vi "FlatToRichcif_pluginloader_DiscoveredPlugin.vi"(5 "OutputClusterType":T1, 11 "InputCluster":T4) -> (3 "OutputCluster":T1)   [LabVIEW 2021, in "CIF_PluginLoader_server.lvlib"]
uses:
  CIF_PluginLoader_server.lvlib
  cif_pluginloader_DiscoveredPlugin_Flat.ctl
  cif_common_Version_Flat.ctl
  cif_management_common_PluginMetadata_Flat.ctl
  cif_pluginloader_DiscoveredPlugin.ctl
  cif_common_Version.ctl
  cif_management_common_PluginMetadata.ctl
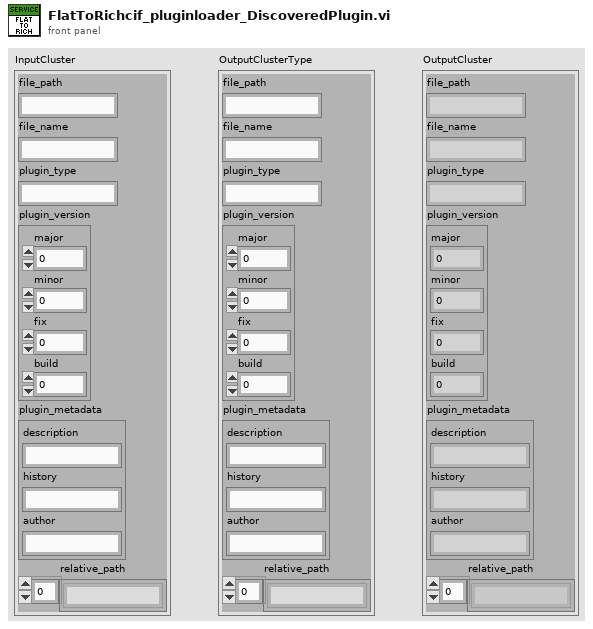
[diagram p1: front panel]
types:
  T1 = typedef "CIF_PluginLoader_server.lvlib/cif_pluginloader_DiscoveredPlugin.ctl" = cluster{"file_path":string, "file_name":string, "plugin_type":string, "plugin_version":T2, "plugin_metadata":T3, "relative_path":string[]}
  T2 = typedef "CIF_PluginLoader_server.lvlib/cif_common_Version.ctl" = cluster{"major":u32, "minor":u32, "fix":u32, "build":u32}
  T3 = typedef "CIF_PluginLoader_server.lvlib/cif_management_common_PluginMetadata.ctl" = cluster{"description":string, "history":string, "author":string}
  T4 = typedef "CIF_PluginLoader_server.lvlib/cif_pluginloader_DiscoveredPlugin_Flat.ctl" = cluster{"file_path":string, "file_name":string, "plugin_type":string, "plugin_version":T5, "plugin_metadata":T6, "relative_path":string[]}
  T5 = typedef "CIF_PluginLoader_server.lvlib/cif_common_Version_Flat.ctl" = cluster{"major":u32, "minor":u32, "fix":u32, "build":u32}
  T6 = typedef "CIF_PluginLoader_server.lvlib/cif_management_common_PluginMetadata_Flat.ctl" = cluster{"description":string, "history":string, "author":string}
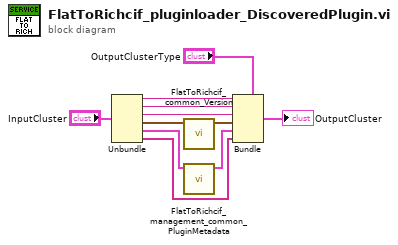
[diagram p0: block diagram]
diagram:
  n1 = Unbundle "Unbundle"("InputCluster") -> ("file_path"=w8:string, "file_name"=w7:string, "plugin_type"=w6:string, "plugin_version"=w5:T5, "plugin_metadata"=w3:T6, "relative_path"=w1:string[])
  n2 = call "FlatToRichcif_common_Version.vi"("InputCluster"=w5) -> ("OutputCluster"=w4:T2)  [unwired: 10 in]
  n3 = call "FlatToRichcif_management_common_PluginMetadata.vi"("InputCluster"=w3) -> ("OutputCluster"=w2:T3)  [unwired: 10 in]
  n4 = Bundle "Bundle"(cluster="OutputClusterType", "file_path"=w8, "file_name"=w7, "plugin_type"=w6, "plugin_version"=w4, "plugin_metadata"=w2, "relative_path"=w1) -> (→"OutputCluster":T1)
